vi "Acqusiton.vi"(8 "error in (no error)":errorcluster) -> (0 "error out":errorcluster, 3 "CanAcqusiton":bool)   [LabVIEW 2014]
uses:
  USBAnalyzerEllisysDll/Debug/USBAnalyzerEllisysDll.dll
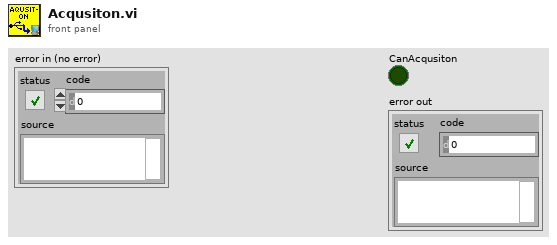
[diagram p1: front panel]
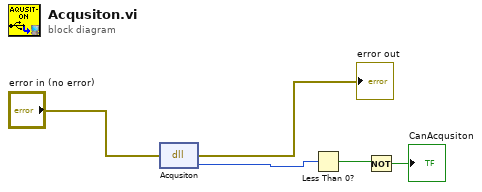
[diagram p0: block diagram]
diagram:
  n1 = dll-call lib="PTH2labs CUsersMichał\tDocumentsEllisysAnalyzerUSBAnalyzerEllisysDllDebugUSBAnalyzerEllisysDll.dll" fn="Acqusiton"(error in="error in (no error)") -> (error out=→"error out":errorcluster, "return type"=w3:i32)  [unwired: 2 in, 1 out]
  n2 = Less Than 0?(x=w3) -> (x < 0?=w2:bool)
  n3 = Not(x=w2) -> (.not. x?=→"CanAcqusiton":bool)
